vi "Stage move.vi"() -> ()   [LabVIEW 2020]
panel:
  out "error out":errorcluster
  in  "Data Collection":T1={"Sample Rate (0: 62.5 mHz)"=0, "Continuous Storage (T: Enable)"=TRUE, "Number of Points (100)"=100, "Channel (1: Channel 1 Display)"=1, "Channel 1 Display (0: X)"=0} {"Channel 1 Display (0: X)" items=["X", "R", "X Noise", "Aux In 1", "Aux In 2"]; "Channel (1: Channel 1 Display)" items=["Channel 1 Display"=1, "Channel 2 Display"=2]; "Sample Rate (0: 62.5 mHz)" items=["62.5 mHz", "125 mHz", "250 mHz", "500 mHz", "1 Hz", "2 Hz", "4 Hz", "8Hz", "16 Hz", "32 Hz", "64 Hz", "128 Hz", "256 Hz", "512 Hz", "Trigger "]}
  in  "Configure":T2={"Lock in Amplifier PORT"="", "Input Connection (0: Single-Ended Voltage) "=0, "Input Coupling (0: AC)"=0, "Input Notch Filter (0: None)"=0, "Reference Source (1: Internal)"=1, "Dynamic Reserve (-1: Auto Reserve)"=-1, "Sensitivity (-1: Auto gain)"=-1, "Time Constant (8: 100ms)"=8} {"Time Constant (8: 100ms)" items=["10 us", "30 us", "100 us", "300 us", "1 ms", "3 ms", "10 ms", "30 ms", "100 ms", "300 ms", "1 s", "3 s", "10 s", "30 s", "100 s", "300 s", "1 ks", "3 ks", "10 ks", "30 ks"]; "Sensitivity (-1: Auto gain)" items=["Auto Gain"=-1, "2 nV/fA"=0, "5 nV/fA"=1, "10 nV/fA"=2, "20 nV/fA"=3, "50 nV/fA"=4, "100 nV/fA"=5, "200 nV/fA"=6, "500 nV/fA"=7, "1 uV/pA"=8, "2 uV/pA"=9, "5 uV/pA"=10, "10 uV/pA"=11, "20 uV/pA"=12, "50 uV/pA"=13, "100 uV/pA"=14, "200 uV/pA"=15, "500 uV/pA"=16, "1 mV/nA"=17, "2 mV/nA"=18, "5 mV/nA"=19, "10 mV/nA"=20, "20 mV/nA"=21, "50 mV/nA"=22, "100 mV/nA"=23, "200 mV/nA"=24, "500 mV/mA"=25, "1 V/uA"=26]; "Dynamic Reserve (-1: Auto Reserve)" items=["Auto Reserve"=-1, "High Reserve"=0, "Normal"=1, "Low Noise"=2]; "Reference Source (1: Internal)" items=["External", "Internal"]; "Input Notch Filter (0: None)" items=["None", "Line Notch", "2x Line Notch", "Both Notch Filters"]; "Input Coupling (0: AC)" items=["AC", "DC"]; "Input Connection (0: Single-Ended Voltage)" items=["Single-Ended Voltage", "Differential Voltage", "1 MOhm Current Gain", "100 MOhm Current Gain"]}
  in  "Stage":T3={"Holmarc Stage"="COM4", "Width"=0, "Step width "=0}
  out "B out":dbl
  out "A out":dbl
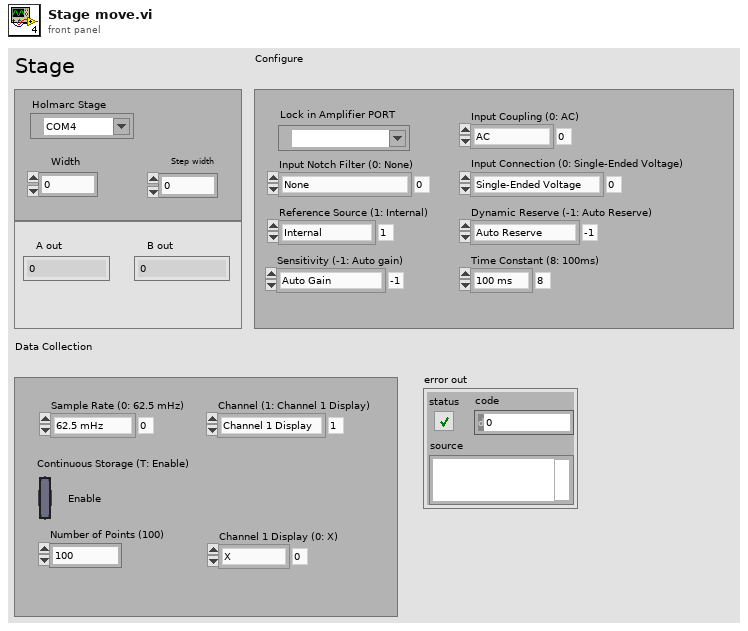
[diagram p1: front panel]
types:
  T1 = cluster{"Sample Rate (0: 62.5 mHz)":u16, "Continuous Storage (T: Enable)":bool, "Number of Points (100)":u32, "Channel (1: Channel 1 Display)":u16, "Channel 1 Display (0: X)":u16}
  T2 = cluster{"Lock in Amplifier PORT":refnum<visa-resource-name>, "Input Connection (0: Single-Ended Voltage) ":u16, "Input Coupling (0: AC)":u16, "Input Notch Filter (0: None)":u16, "Reference Source (1: Internal)":u16, "Dynamic Reserve (-1: Auto Reserve)":i16, "Sensitivity (-1: Auto gain)":i16, "Time Constant (8: 100ms)":u16}
  T3 = cluster{"Holmarc Stage":refnum<visa-resource-name>, "Width":i32, "Step width ":i32}
  T4 = cluster{"Number of Points (100)":u32, "VISA resource name out":refnum<visa-resource-name>, "Channel (1: Channel 1 Display)":u16, "error out":errorcluster}
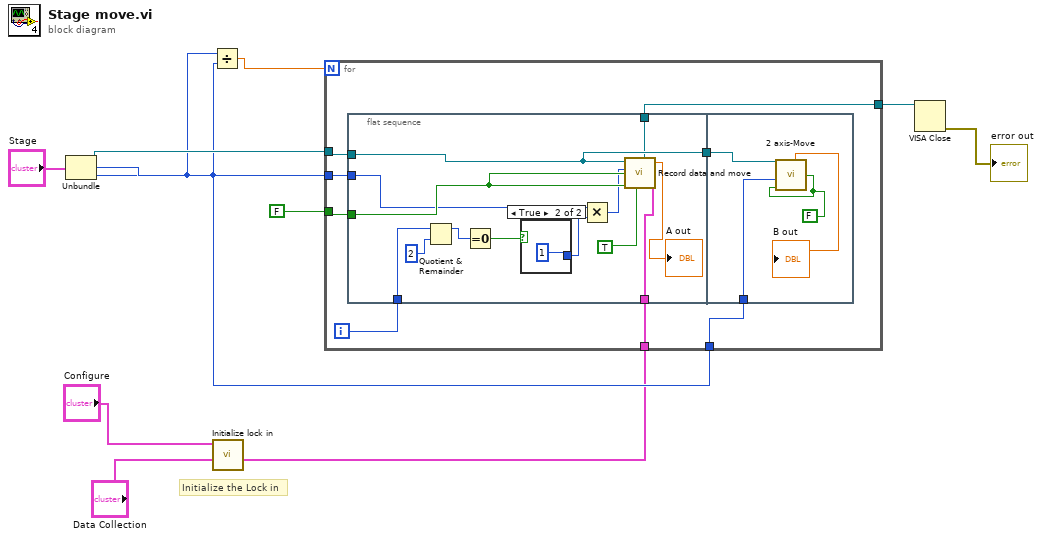
[diagram p0: block diagram]
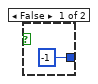
[diagram p2: hidden frame]
diagram:
  # "Initialize the Lock in"
  n1 = Unbundle("Stage") -> ("Holmarc Stage"=w8:refnum<visa-resource-name>, "Width"=w7:i32, "Step width"=w6:i32)
  n2 = Divide(x=w7, y=w6) -> (x/y=w10:dbl)
  n3 = call "Initialize lock in.vi"("Data Collection"="Data Collection", "Configure"="Configure") -> ("Output"=w3:T4)  [unwired: 9 in]
  n4 = for {
    N: w10 -> [_]
    tunnel: w8 -> [w19]
    tunnel: FALSE ("Accelaration") -> [w18]
    tunnel: w7 -> [w16]
    tunnel: w6 -> [w14]
    tunnel: w3 -> [w13]
    tunnel: [w12] -> w2
    i -> [w17]
    n5 = flat-sequence {
      tunnel: w19 -> [w24]
      tunnel: w18 -> [w32]
      tunnel: w17 -> [w31]
      tunnel: w16 -> [w27]
      tunnel: [w24] -> w15
      tunnel: w13 -> [w21]
      tunnel: [w20] -> w12
      tunnel: w15 -> [w38]
      tunnel: w14 -> [w37]
      frame #0 {
        n6 = Quotient & Remainder(x=w31, y=2) -> (x-y*floor(x/y)=w29:i32)  [unwired: 1 out]
        n7 = Equal To 0?(x=w29) -> (x = 0?=w28:bool)
        n8 = case shown="True" w28 {
          tunnel: [-1 1] -> w26
          frame False {
          }
          frame True {
          }
        }
        n9 = Multiply(x=w27, y=w26) -> (x*y=w25:i32)
        n10 = call "Record data and move.vi"("Lock in Input"=w21, "Deceleration"=w32, "RESET"=TRUE, "Accelaration"=w32, "A axis"=w25, "Comport"=w24) -> ("A out"=→"A out":dbl, "VISA resource name out"=w20:refnum<visa-resource-name>)  [unwired: 3 in]
      }
      frame #1 {
        w36 = FALSE ("Deceleration")
        n11 = call "2 axis-Move.vi"("Deceleration"=w36, "Accelaration"=w36, "B axis"=w37, "Comport"=w38) -> ("B out"=→"B out":dbl)  [unwired: 5 in, 1 out]
      }
    }
  }
  n12 = VISA Close(VISA resource name=w2) -> (error out=→"error out":errorcluster)  [unwired: 1 in]
